vi "Close.vi"(8 "error in (no error)":errorcluster) -> (0 "error out":errorcluster)   [LabVIEW 2023, in "HighFinesse WS5.lvlib"]
doc: "Closes the wavelength meter program.\n\nDoes not work properly. Redone to bring up WLM to force user to close it manually. --David"
uses:
  HighFinesse WS5.lvlib
  Variable Typedefs.llb/WLM control mode.ctl
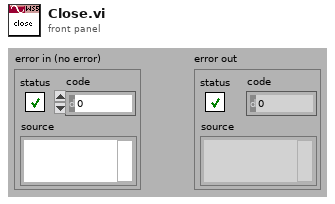
[diagram p1: front panel]
types:
  T1 = typedef "HighFinesse WS5.lvlib/WLM control mode.ctl" = i16
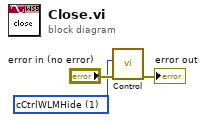
[diagram p0: block diagram]
diagram:
  w1 = T1 1 items=["cCtrlWLMShow", "cCtrlWLMHide", "cCtrlWLMExit"] ("WLM Control Mode Constants")
  n1 = call "Control.vi"("error in (no error)"="error in (no error)", "command (show)"=w1) -> ("error out"=→"error out":errorcluster)  [unwired: 9 out]
